vi "WPI_CameraGet Image From HTTP.vi"(8 "error in (no error)":errorcluster, 9 "Unflatten":bool, 10 "Image In":T1, 11 "connection ID":refnum<k5>) -> (0 "error out":errorcluster, 1 "Size":i32, 2 "Image Out":T1, 3 "connection ID (dup)":refnum<k5>)   [LabVIEW 2017]
doc: "This software is licensed. Open the labview\\readme\\WPI Robotics Library Open Source License.txt file for more information."
uses:
  <vilib>/vision/Image Controls.llb/IMAQ Image.ctl
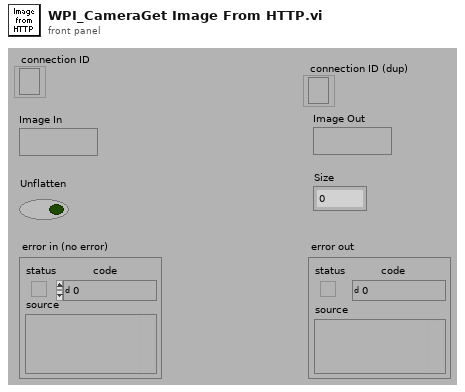
[diagram p1: front panel]
types:
  T1 = typedef "IMAQ Image.ctl" = refnum<image>
  T2 = enum16{"Standard", "Buffered", "CRLF", "Immediate"}
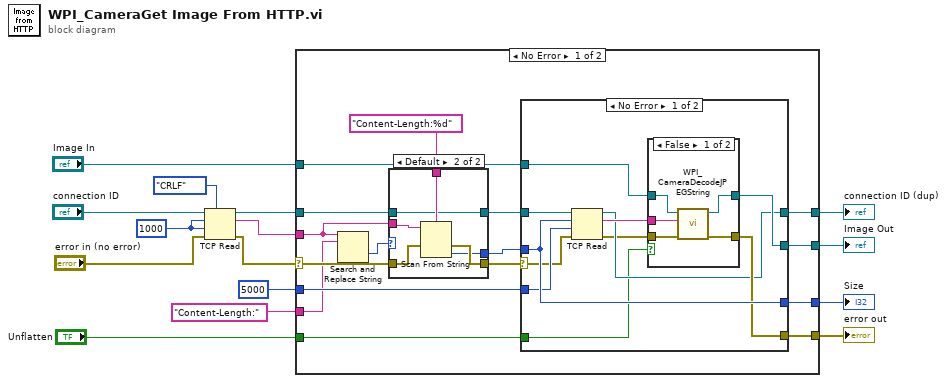
[diagram p0: block diagram]
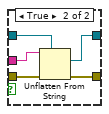
[diagram p3: hidden frame]
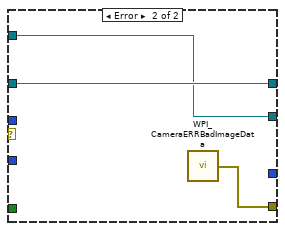
[diagram p4: hidden frame]
diagram:
  w3 = 1000 ("bytes to read")
  n1 = TCP Read(connection ID="connection ID", bytes to read=w3, error in (no error)="error in (no error)", 7:T2."CRLF" ("mode (standard)"), 9:w3) -> (connection ID out=w15:refnum<k5>, data out=w12:string, error out=w7:errorcluster)
  n2 = case shown="No Error" w7 {
    selector: w7 -> [w24 w64]
    tunnel: w15 -> [w26 w66]
    tunnel: "Image In" -> [w31 w65]
    tunnel: w12 -> [w20 _]
    tunnel: [w30 w64] -> w10
    tunnel: [w29 w65] -> w9
    tunnel: [w28 w66] -> w8
    tunnel: [w27 _] -> w6
    tunnel: "Content-Length:" ("regular expression") -> [w19 _]
    tunnel: "Unflatten" -> [w21 _]
    tunnel: 5000 ("bytes to read") -> [w22 _]
    frame No Error {
      n3 = Search and Replace String(input string=w20, search string=w19) -> (offset past replacement=w18:i32)  [unwired: 1 in, 8 out]
      n4 = case shown="Default" w18 {
        tunnel: w26 -> [w33 w37]
        tunnel: [w33 w37] -> w25
        tunnel: w24 -> [w32 w36]
        tunnel: [w32 w35] -> w23
        tunnel: w20 -> [_ w39]
        tunnel: "Content-Length:%d" ("regular expression") -> [_ w38]
        tunnel: [_ w34] -> w16
        frame 0 {
        }
        frame Default {
          n5 = Scan From String(format string=w38, input string=w39, error in=w36) -> (error out=w35:errorcluster, output 1=w34:i32)  [unwired: 1 in, 3 out]
        }
      }
      n6 = case shown="No Error" w23 {
        selector: w23 -> [w45 _]
        tunnel: w25 -> [w50 w63]
        tunnel: w31 -> [w47 w62]
        tunnel: [w44 w61] -> w30
        tunnel: [w46 w62] -> w29
        tunnel: [w42 w63] -> w28
        tunnel: [w49 _] -> w27
        tunnel: w16 -> [w49 _]
        tunnel: w22 -> [w48 _]
        tunnel: w21 -> [w41 _]
        frame No Error {
          n7 = TCP Read(connection ID=w50, bytes to read=w49, error in (no error)=w45, 9:w48) -> (connection ID out=w42:refnum<k5>, data out=w43:string, error out=w40:errorcluster)  [unwired: 1 out]
          n8 = case shown="False" w41 {
            tunnel: w47 -> [w55 w59]
            tunnel: [w54 w60] -> w46
            tunnel: w43 -> [w53 w57]
            tunnel: [w52 w58] -> w44
            tunnel: w40 -> [w51 w56]
            frame False {
              n9 = call <vilib>:"WPI_CameraDecodeJPEGString.vi"("error in"=w51, "Compressed Image"=w53, "Image In"=w55) -> ("error out"=w52:errorcluster, "Image Out"=w54:T1)  [unwired: 3 out]
            }
            frame True {
              n10 = Unflatten From String(type=w59, binary string=w57, error in (no error)=w56) -> (value=w60:T1, error out=w58:errorcluster)  [unwired: 2 in, 1 out]
            }
          }
        }
        frame Error {
          n11 = call <vilib>:"WPI_CameraERRBadImageData.vi"() -> ("error out"=w61:errorcluster)
        }
      }
    }
    frame Error {
    }
  }
  "error out" <- w10
  "Image Out" <- w9
  "connection ID (dup)" <- w8
  "Size" <- w6
